vi "Meter Test.vi"(8 "error in":errorcluster, 11 "IED Test in":refnum<class "IED Test.lvclass">) -> (0 "error out":errorcluster, 2 "Test Result":T1=enum."Success", 3 "IED Test out":refnum<class "IED Test.lvclass">)   [LabVIEW 2018, in "IED Test Framework.lvlib" / "IED Test.lvclass"]
uses:
  IED Test.lvclass
  C:/Program Files (x86)/National Instruments/LabVIEW 2018/vi.lib/ActorFramework/Actor/Actor.lvclass
  C:/Users/Administrator/Desktop/2018LabVIEW EMS/EMS Generic Actor/EMS Generic/EMS Generic.lvclass
  Controls/Test Result.ctl
  <vilib>/ORNL/CSEISMIC DDS/CSEISMIC DDS Base/Data Types/Controls/DeviceClass Selector.ctl
  Meter Actor/Meter/Meter.lvclass
  C:/Users/Administrator/Desktop/2018LabVIEW EMS/IED Actors/Device DDS Communications Framework/Device DDS Communications/Device DDS Communications.lvclass
  <vilib>/ORNL/CSEISMIC DDS/CSEISMIC DDS Base/CSEISMIC DDS.lvclass/CSEISMIC DDS.ctl
  <vilib>/ORNL/CSEISMIC DDS/CSEISMIC DDS Base/Data Types/Controls/DeviceID.ctl
  <vilib>/ActorFramework/Message Enqueuer/Message Enqueuer.lvclass/Message Enqueuer.ctl
  <vilib>/ORNL/CSEISMIC DDS/CSEISMIC DDS Base/Accessors/Write DDS Reference.vi
  <vilib>/ORNL/CSEISMIC DDS/CSEISMIC DDS Base/Accessors/Read DDS Reference.vi
  <vilib>/ActorFramework/Message Enqueuer/Enqueue.vi
  <vilib>/ORNL/CSEISMIC DDS/DDS Writer/DDS Writer.lvclass
  C:/Program Files (x86)/National Instruments/LabVIEW 2018/vi.lib/ORNL/CSEISMIC DDS/CSEISMIC DDS Base/CSEISMIC DDS.lvclass
  <vilib>/ActorFramework/Stop Msg/Stop Msg.lvclass
  C:/Program Files (x86)/National Instruments/LabVIEW 2018/vi.lib/ActorFramework/Message/Message.lvclass
  <vilib>/ORNL/CSEISMIC DDS/CSEISMIC DDS Base/Error Handler.vi
  <vilib>/ActorFramework/Message Priority Queue/Priority Enqueue.vi
  <vilib>/ORNL/CSEISMIC DDS/CSEISMIC DDS Base/CSEISMIC DDS.lvclass
  Device DDS Communications Framework/Device DDS Communications/Device DDS Communications.lvclass
  <vilib>/ActorFramework/Actor/Actor.lvclass
  EMS Generic Actor/EMS Generic/EMS Generic.lvclass
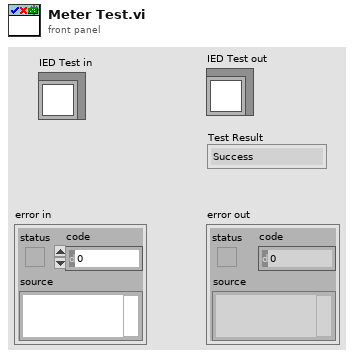
[diagram p1: front panel]
types:
  T1 = typedef "IED Test Framework.lvlib/IED Test.lvclass/Test Result.ctl" = enum16{"Invalid", "Success", "Failure", "Error", "Timeout"}
  T2 = typedef "CSEISMIC DDS.lvlib/CSEISMIC DDS.lvclass/DeviceID.ctl" = string
  T3 = typedef "CSEISMIC DDS.lvlib/CSEISMIC DDS.lvclass/DeviceClass Selector.ctl" = u16
  T4 = typedef "CSEISMIC DDS.lvlib/CSEISMIC DDS.lvclass/Meter_Measurement.ctl" = cluster{"DeviceID":T2, "Voltage":dbl[], "Current":dbl[], "RealPower":dbl[], "ReactivePower":dbl[], "LineConfig":u8[], "Frequency":dbl}
  T5 = typedef "CSEISMIC DDS.lvlib/CSEISMIC DDS.lvclass/Meter_Info.ctl" = cluster{"DeviceID":T2, "LineConfig":u8[], "NominalVoltage(V)":dbl}
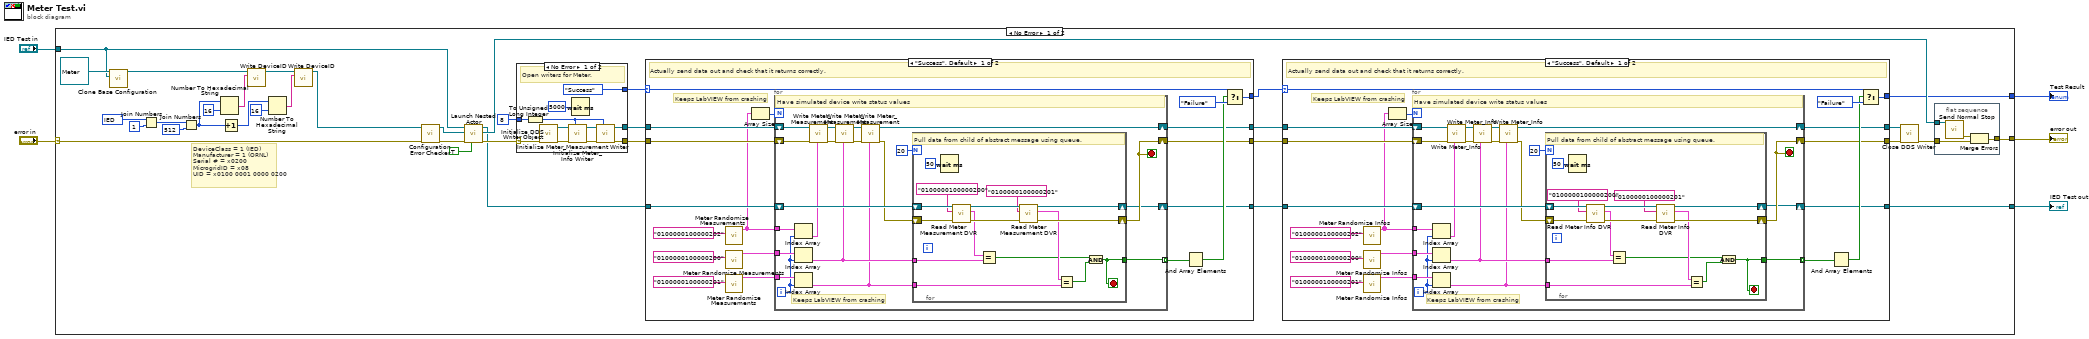
[diagram p0: block diagram]
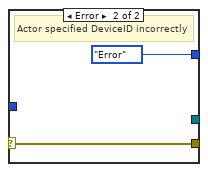
[diagram p3: hidden frame]
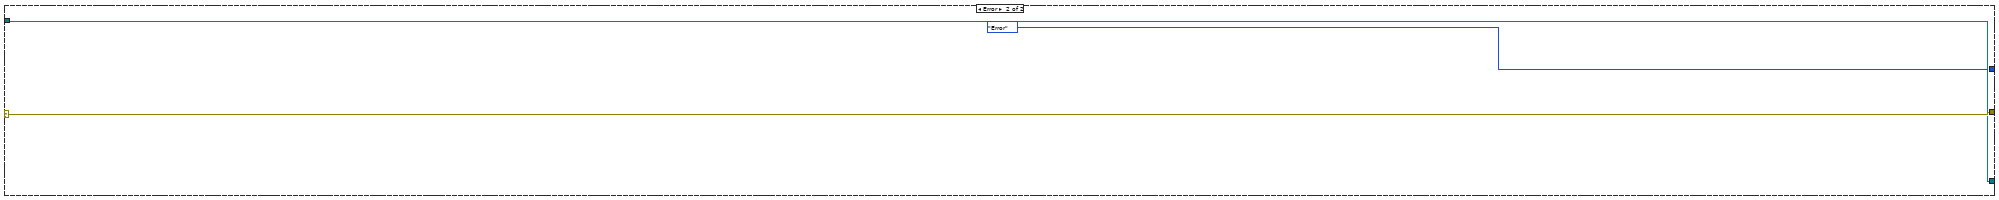
[diagram p5: hidden frame]
diagram:
  n1 = case shown="No Error" "error in" {
    selector: "error in" -> [w37 w177]
    tunnel: [w39 w177] -> w5
    tunnel: [w6 w176] -> w3
    tunnel: "IED Test in" -> [w9 w176]
    tunnel: [w13 Test_Result."Error" ("f")] -> w4
    frame No Error {
      w30 = T3 256 items=["Invalid"=0, "IED"=256, "DER"=512, "Relay"=768, "Meter"=1024, "Load"=1280, "Forecast"=1536, "Price"=1792, "Energy Storage"=513, "PV"=514, "Generator"=515, "Smart Relay"=769, "PCC"=770, "Smart Meter"=1025, "PMU"=1026, "HVAC"=1281] ("DeviceClass")
      # "DeviceClass = 1 (IED)\nManufacturer = 1 (ORNL)\nSerial # = x0200\nMicrogridID = x08\nUID = x0100 0001 0000 0200"
      n2 = call-dynamic "Clone Base Configuration.vi"("Source Object"=w9, "Target Object in"=refnum<class "Meter.lvclass"> refnum ("Meter Actor.lvlib:Meter.lvclass")) -> ("Target Object out"=w11:refnum<class "Meter.lvclass">)  [unwired: 9 in]
      n3 = Join Numbers(hi=w30, lo=u16 1 ("MicrogridID")) -> ((hi.lo)=w27:u32)
      n4 = Join Numbers(hi=w27, lo=u32 512 ("MicrogridID")) -> ((hi.lo)=w32:u64)
      n5 = Number To Hexadecimal String(1:i16 16 ("width (-)"), 2:w32) -> (0:w25:string)
      n6 = Increment(x=w32) -> (x+1=w34:u64)
      n7 = call-dynamic "Write DeviceID.vi"("DeviceID"=w25, "Device DDS Communications in"=w11) -> ("Device DDS Communications out"=w29:refnum<class "Meter.lvclass">)  [unwired: 9 in]
      n8 = Number To Hexadecimal String(1:i16 16 ("width (-)"), 2:w34) -> (0:w35:string)
      n9 = call-dynamic "Write DeviceID.vi"("DeviceID"=w35, "Device DDS Communications in"=w29) -> ("Device DDS Communications out"=w12:refnum<class "Meter.lvclass">)  [unwired: 9 in]
      n10 = call "Configuration Error Checker.vi"("error in"=w37, "Device DDS Communications in"=w12) -> ("error out"=w40:errorcluster, "Device DDS Communications out"=w38:refnum<class "Meter.lvclass">)  [unwired: 8 in]
      n11 = call <vilib>:"Launch Nested Actor.vi"("Open Actor Core front panel? (F)"=TRUE, "error in (no error)"=w40, "Nested Actor"=w38, "Caller Actor in"=w9) -> ("error out"=w23:errorcluster, "Nested Actor's Enqueuer"=w36:refnum<class "Message Enqueuer.lvclass">, "Caller Actor out"=w7:refnum<class "IED Test.lvclass">)  [unwired: 5 in]
      n12 = case shown="No Error" w23 {
        selector: w23 -> [w112 w116]
        tunnel: [w105 w116] -> w20
        tunnel: u32 8 ("domain id") -> [w114 _]
        tunnel: [Test_Result."Success" ("Test Result in") Test_Result."Error" ("Test Result")] -> w22
        tunnel: [w104 _] -> w21
        frame No Error {
          # "Open writers for Meter."
          n13 = To Unsigned Long Integer(number=w114) -> (unsigned 32bit integer=w107:u32)
          n14 = call <vilib>:"Initialize DDS Writer Object.vi"("error in"=w112) -> ("error out"=w111:errorcluster, "DDS Writer out"=w110:refnum<class "DDS Writer.lvclass">)  [unwired: 9 in]
          n15 = call <vilib>:"Initialize Meter_Info Writer.vi"("MicrogridID"=w107, "error in"=w111, "DDS Writer in"=w110) -> ("error out"=w108:errorcluster, "DDS Writer out"=w109:refnum<class "DDS Writer.lvclass">)  [unwired: 7 in]
          n16 = Wait (ms)(milliseconds to wait=u32 5000) -> ()  [unwired: 1 out]
          n17 = call <vilib>:"Initialize Meter_Measurement Writer.vi"("MicrogridID"=w107, "error in"=w108, "DDS Writer in"=w109) -> ("error out"=w105:errorcluster, "DDS Writer"=w104:refnum<class "DDS Writer.lvclass">)  [unwired: 7 in]
        }
        frame Error {
          # "Actor specified DeviceID incorrectly"
        }
      }
      n18 = case shown="\"Success\", Default" w22 {
        selector: w22 -> [w62 w102]
        tunnel: w21 -> [w63 w101]
        tunnel: w7 -> [w57 w100]
        tunnel: w20 -> [w58 w103]
        tunnel: [w60 w102] -> w17
        tunnel: [w56 w103] -> w18
        tunnel: [w54 w101] -> w19
        tunnel: [w46 w100] -> w8
        frame "Success", Default {
          # "Keeps LabVIEW from crashing"
          # "Actually send data out and check that it returns correctly."
          n19 = call "Meter Randomize Measurements.vi"("DeviceID"=T2 "0100000100000202" ("(hi.lo)")) -> ("Meter_Measurement Array out"=w53:T4[])  [unwired: 10 in]
          n20 = call "Meter Randomize Measurements.vi"("DeviceID"=T2 "0100000100000200" ("(hi.lo)")) -> ("Meter_Measurement Array out"=w48:T4[])  [unwired: 10 in]
          n21 = call "Meter Randomize Measurements.vi"("DeviceID"=T2 "0100000100000201" ("(hi.lo)")) -> ("Meter_Measurement Array out"=w49:T4[])  [unwired: 10 in]
          n22 = Array Size(array=w53) -> (size(s)=w55:i32)
          n23 = for {
            N: w55 -> [_]
            shift-right: [w80] -> w54
            shift-left: w63 -> [w83]
            tunnel: w53 -> [w76]
            tunnel: w49 -> [w71]
            tunnel: w48 -> [w72]
            shift-right: [w73] -> w56
            shift-left: w58 -> [w79]
            tunnel: [w67] -> w47 mode=indexing
            shift-right: [w64] -> w46
            shift-left: w57 -> [w75]
            i -> [w69]
            stop <- w73 stop-if-true
            # "Keeps LabVIEW from crashing"
            # "Have simulated device write status values"
            n24 = Index Array(array=w76, index=w69) -> (element=w68:T4)
            n25 = Index Array(array=w72, index=w69) -> (element=w66:T4)
            n26 = Index Array(array=w71, index=w69) -> (element=w65:T4)
            n27 = call <vilib>:"Write Meter_Measurement.vi"("Meter_Measurement"=w68, "error in"=w79, "DDS Writer in"=w83) -> ("error out"=w78:errorcluster, "DDS Writer out"=w82:refnum<class "DDS Writer.lvclass">)  [unwired: 7 in]
            n28 = call <vilib>:"Write Meter_Measurement.vi"("Meter_Measurement"=w66, "error in"=w78, "DDS Writer in"=w82) -> ("error out"=w77:errorcluster, "DDS Writer out"=w81:refnum<class "DDS Writer.lvclass">)  [unwired: 7 in]
            n29 = call <vilib>:"Write Meter_Measurement.vi"("Meter_Measurement"=w65, "error in"=w77, "DDS Writer in"=w81) -> ("error out"=w74:errorcluster, "DDS Writer out"=w80:refnum<class "DDS Writer.lvclass">)  [unwired: 7 in]
            n30 = for {
              N: 20 -> [_]
              shift-right: [w92] -> w73
              shift-left: w74 -> [w99]
              tunnel: [w91] -> w67
              tunnel: w66 -> [w89]
              tunnel: w65 -> [w88]
              shift-right: [w84] -> w64
              shift-left: w75 -> [w98]
              stop <- w91 stop-if-true
              # "Pull data from child of abstract message using queue."
              n31 = Wait (ms)(milliseconds to wait=u32 50) -> ()  [unwired: 1 out]
              n32 = call "Read Meter Measurement DVR.vi"("error in"=w99, "DeviceID"=T2 "0100000100000200" ("(hi.lo)"), "EMS Generic in"=w98) -> ("error out"=w97:errorcluster, "Meter_Measurement"=w90:T4, "EMS Generic out"=w96:refnum<class "IED Test.lvclass">)  [unwired: 5 in, 1 out]
              n33 = Equal?(x=w90, y=w89) -> (x = y?=w85:bool)
              n34 = call "Read Meter Measurement DVR.vi"("error in"=w97, "DeviceID"=T2 "0100000100000201" ("(hi.lo)"), "EMS Generic in"=w96) -> ("error out"=w92:errorcluster, "Meter_Measurement"=w87:T4, "EMS Generic out"=w84:refnum<class "IED Test.lvclass">)  [unwired: 5 in, 1 out]
              n35 = Equal?(x=w87, y=w88) -> (x = y?=w86:bool)
              n36 = And(x=w85, y=w86) -> (x .and. y?=w91:bool)
            }
          }
          n37 = And Array Elements(Boolean array=w47) -> (logical AND=w59:bool)
          n38 = Select(t=w62, s=w59, f=Test_Result."Failure") -> (s? t:f=w60:T1)
        }
        frame "Error" {
        }
      }
      n39 = case shown="\"Success\", Default" w17 {
        selector: w17 -> [w133 w173]
        tunnel: w19 -> [w134 w172]
        tunnel: w8 -> [w128 w171]
        tunnel: w18 -> [w129 w174]
        tunnel: [w131 w173] -> w13
        tunnel: [w127 w174] -> w15
        tunnel: [w125 w172] -> w16
        tunnel: [w118 w171] -> w6
        frame "Success", Default {
          # "Keeps LabVIEW from crashing"
          # "Actually send data out and check that it returns correctly."
          n40 = call "Meter Randomize Infos.vi"("DeviceID"=T2 "0100000100000202" ("(hi.lo)")) -> ("Meter_Info Array out"=w124:T5[])  [unwired: 10 in]
          n41 = call "Meter Randomize Infos.vi"("DeviceID"=T2 "0100000100000200" ("(hi.lo)")) -> ("Meter_Info Array out"=w119:T5[])  [unwired: 10 in]
          n42 = call "Meter Randomize Infos.vi"("DeviceID"=T2 "0100000100000201" ("(hi.lo)")) -> ("Meter_Info Array out"=w120:T5[])  [unwired: 10 in]
          n43 = Array Size(array=w124) -> (size(s)=w126:i32)
          n44 = for {
            N: w126 -> [_]
            shift-right: [w151] -> w125
            shift-left: w134 -> [w154]
            tunnel: w124 -> [w147]
            tunnel: w120 -> [w142]
            tunnel: w119 -> [w143]
            shift-right: [w144] -> w127
            shift-left: w129 -> [w150]
            shift-right: [w138] -> w118
            shift-left: w128 -> [w146]
            tunnel: [w135] -> w117 mode=indexing
            i -> [w140]
            stop <- w144 stop-if-true
            # "Keeps LabVIEW from crashing"
            # "Have simulated device write status values"
            n45 = Index Array(array=w147, index=w140) -> (element=w139:T5)
            n46 = Index Array(array=w143, index=w140) -> (element=w137:T5)
            n47 = Index Array(array=w142, index=w140) -> (element=w136:T5)
            n48 = call <vilib>:"Write Meter_Info.vi"("Meter_Info"=w139, "error in"=w150, "DDS Writer in"=w154) -> ("error out"=w149:errorcluster, "DDS Writer out"=w153:refnum<class "DDS Writer.lvclass">)  [unwired: 7 in]
            n49 = call <vilib>:"Write Meter_Info.vi"("Meter_Info"=w137, "error in"=w149, "DDS Writer in"=w153) -> ("error out"=w148:errorcluster, "DDS Writer out"=w152:refnum<class "DDS Writer.lvclass">)  [unwired: 7 in]
            n50 = call <vilib>:"Write Meter_Info.vi"("Meter_Info"=w136, "error in"=w148, "DDS Writer in"=w152) -> ("error out"=w145:errorcluster, "DDS Writer out"=w151:refnum<class "DDS Writer.lvclass">)  [unwired: 7 in]
            n51 = for {
              N: 20 -> [_]
              shift-right: [w167] -> w144
              shift-left: w145 -> [w169]
              shift-right: [w162] -> w138
              shift-left: w146 -> [w166]
              tunnel: w137 -> [w160]
              tunnel: w136 -> [w158]
              tunnel: [w155] -> w135
              stop <- w155 stop-if-true
              # "Pull data from child of abstract message using queue."
              n52 = Wait (ms)(milliseconds to wait=u32 50) -> ()  [unwired: 1 out]
              n53 = call "Read Meter Info DVR.vi"("error in"=w169, "DeviceID"=T2 "0100000100000200" ("(hi.lo)"), "EMS Generic in"=w166) -> ("error out"=w168:errorcluster, "Meter_Info"=w161:T5, "EMS Generic out"=w165:refnum<class "IED Test.lvclass">)  [unwired: 5 in, 1 out]
              n54 = Equal?(x=w161, y=w160) -> (x = y?=w157:bool)
              n55 = call "Read Meter Info DVR.vi"("error in"=w168, "DeviceID"=T2 "0100000100000201" ("(hi.lo)"), "EMS Generic in"=w165) -> ("error out"=w167:errorcluster, "Meter_Info"=w159:T5, "EMS Generic out"=w162:refnum<class "IED Test.lvclass">)  [unwired: 5 in, 1 out]
              n56 = Equal?(x=w159, y=w158) -> (x = y?=w156:bool)
              n57 = And(x=w157, y=w156) -> (x .and. y?=w155:bool)
            }
          }
          n58 = And Array Elements(Boolean array=w117) -> (logical AND=w130:bool)
          n59 = Select(t=w133, s=w130, f=Test_Result."Failure") -> (s? t:f=w131:T1)
        }
        frame "Error" {
        }
      }
      n60 = call <vilib>:"Close DDS Writer.vi"("error in"=w15, "DDS Writer in"=w16) -> ("error out"=w14:errorcluster)  [unwired: 9 in]
      n61 = flat-sequence {
        tunnel: w36 -> [w45]
        tunnel: [w43] -> w39
        tunnel: w14 -> [w42]
        frame #0 {
          n62 = call <vilib>:"Send Normal Stop.vi"("Message Enqueuer"=w45) -> ("error out"=w44:errorcluster)  [unwired: 10 in]
          n63 = Merge Errors(w44, w42) -> (w43:errorcluster)
        }
      }
    }
    frame Error {
    }
  }
  "error out" <- w5
  "IED Test out" <- w3
  "Test Result" <- w4
